vi "Remakejh.vi"   [LabVIEW 2015]
uses:
  <vilib>/NXT/Block Support/NXT_InputPort.ctl
  <vilib>/NXT/Block Support/NXT_OutputPort.ctl
  <vilib>/NXT/Dual Mode Library/Sensors/Light_On.vi
  <vilib>/NXT/Dual Mode Library/Sensors/Sonar_cm.vi
  <vilib>/NXT/NXTIO Xnodes/NXTIONodeSubVIs/NXTMoveMotors.vi
  <vilib>/NXT/Dual Mode Library/Waits/Wait_Num(msec).vi
  <vilib>/NXT/Subs/LVHSConnector.ctl
  <vilib>/NXT/NXTIO Xnodes/AddressXNode/NXTIOAddress.xnode
  <vilib>/NXT/NXTIO Xnodes/NXTIOXNode/NXTIO.xnode
  <vilib>/NXT/LegoClasses/BrickReference/BrickReference.lvclass
types:
  T1 = typedef "NXT_OutputPort.ctl" = u8
  T2 = typedef "NXT_InputPort.ctl" = u32
  T3 = typedef "LVHSConnector.ctl" = refnum<class "BrickReference.lvclass">
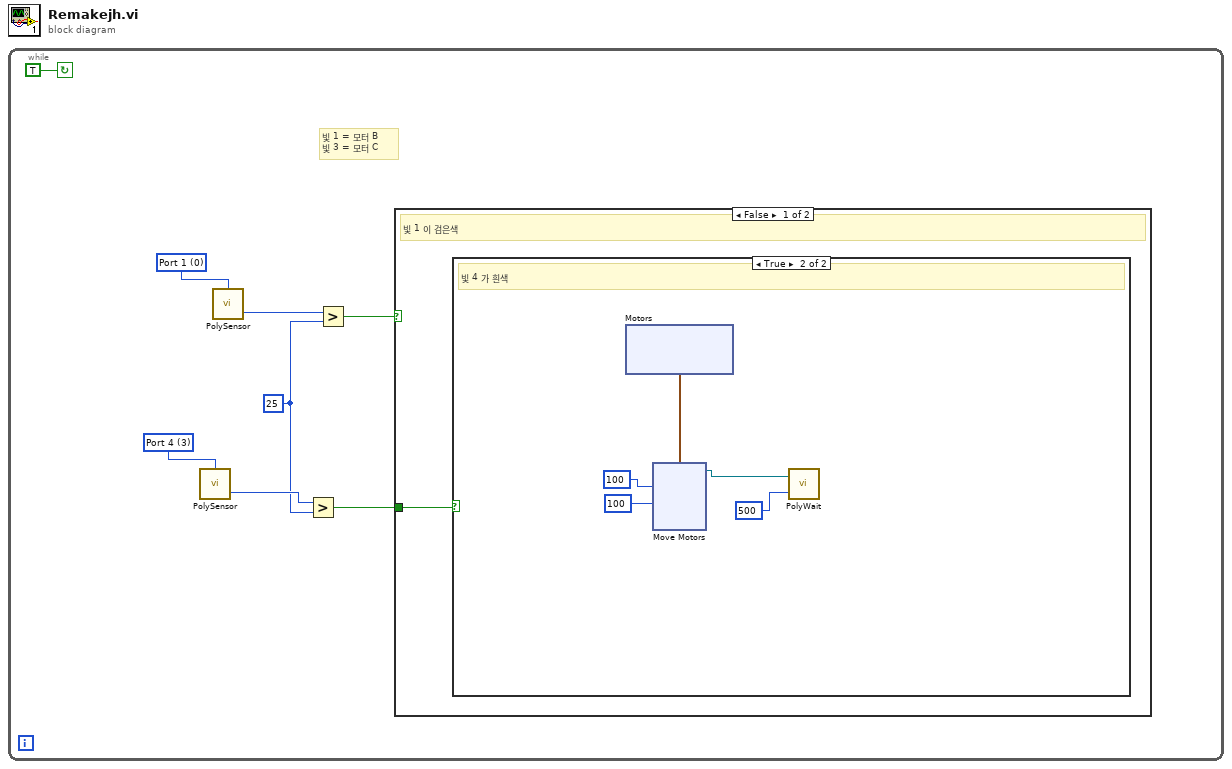
[diagram p0: block diagram]
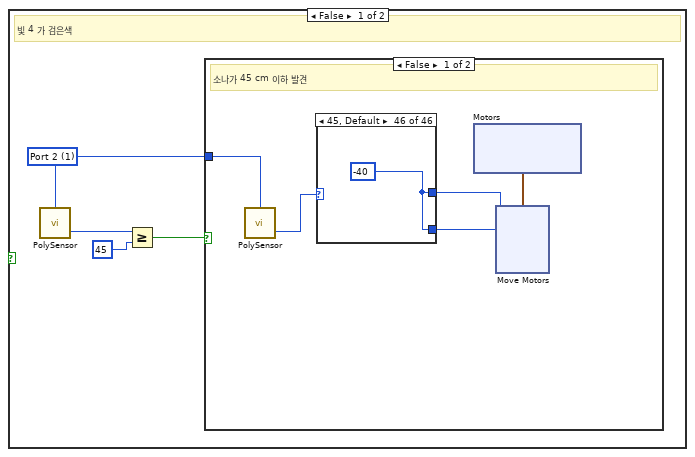
[diagram p2: hidden frame]
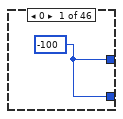
[diagram p3: hidden frame]
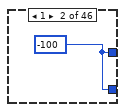
[diagram p4: hidden frame]
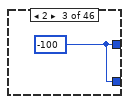
[diagram p5: hidden frame]
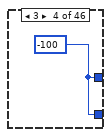
[diagram p6: hidden frame]
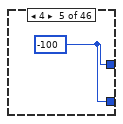
[diagram p7: hidden frame]
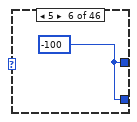
[diagram p8: hidden frame]
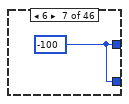
[diagram p9: hidden frame]
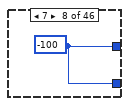
[diagram p10: hidden frame]
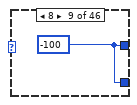
[diagram p11: hidden frame]
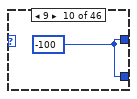
[diagram p12: hidden frame]
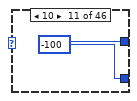
[diagram p13: hidden frame]
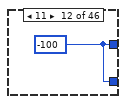
[diagram p14: hidden frame]
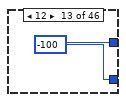
[diagram p15: hidden frame]
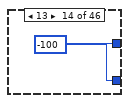
[diagram p16: hidden frame]
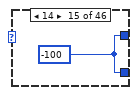
[diagram p17: hidden frame]
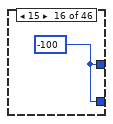
[diagram p18: hidden frame]
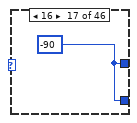
[diagram p19: hidden frame]
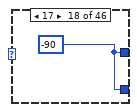
[diagram p20: hidden frame]
diagram:
  n1 = while {
    stop <- TRUE continue-if-true
    w1 = i16 25 ("y")
    w6 = T2 0 items=["Port 1", "Port 2", "Port 3", "Port 4"] ("Port (Port 3)")
    w5 = T2 3 items=["Port 1", "Port 2", "Port 3", "Port 4"] ("Port (Port 3)")
    # "빛 1 = 모터 B\n빛 3 = 모터 C"
    n2 = call-poly <vilib>:"PolySensor.vi"("Port (Port 3)"=w5) -> ("Scaled Value"=w7:i16)  [unwired: 2 in, 1 out]
    n3 = call-poly <vilib>:"PolySensor.vi"("Port (Port 3)"=w6) -> ("Scaled Value"=w8:i16)  [unwired: 2 in, 1 out]
    n4 = Greater?(x=w7, y=w1) -> (0:w3:bool)
    n5 = Greater?(x=w8, y=w1) -> (0:w4:bool)
    n6 = case shown="False" w4 {
      tunnel: w3 -> [w9 w122]
      frame False {
        # "빛 1 이 검은색"
        n7 = case shown="True" w9 {
          frame False {
            w10 = T2 1 items=["Port 1", "Port 2", "Port 3", "Port 4"] ("Port (Port 4)")
            # "빛 4 가 검은색"
            n8 = call-poly <vilib>:"PolySensor.vi"("Port (Port 4)"=w10) -> ("Distance (cm)"=w13:i16)  [unwired: 2 in, 1 out]
            n9 = Greater Or Equal?(x=w13, y=i16 45) -> (x >= y?=w11:bool)
            n10 = case shown="False" w11 {
              tunnel: w10 -> [w18 _]
              frame False {
                # "소나가 45 cm 이하 발견"
                n11 = call-poly <vilib>:"PolySensor.vi"("Port (Port 4)"=w18) -> ("Distance (cm)"=w17:i16)  [unwired: 2 in, 1 out]
                n12 = case shown="45, Default" w17 {
                  tunnel: [w28 w29 w30 w31 w32 w33 w34 w35 w36 w37 w38 w39 w40 w41 w42 w43 w44 w45 w46 w47 w48 w49 w50 w51 w52 w53 w54 w55 w56 w57 w58 w59 w60 w61 w62 w63 w64 w65 w66 w67 w68 w69 w70 w71 w72 w73] -> w15
                  tunnel: [w28 w29 w30 w31 w32 w33 w34 w35 w36 w37 w38 w39 w40 w41 w42 w43 w44 w45 w46 w47 w48 w49 w50 w51 w52 w53 w54 w55 w56 w57 w58 w59 w60 w61 w62 w63 w64 w65 w66 w67 w68 w69 w70 w71 w72 w73] -> w14
                  frame 0 {
                    w28 = i16 -100 ("y")
                  }
                  frame 1 {
                    w29 = i16 -100 ("y")
                  }
                  frame 2 {
                    w30 = i16 -100 ("y")
                  }
                  frame 3 {
                    w31 = i16 -100 ("y")
                  }
                  frame 4 {
                    w32 = i16 -100 ("y")
                  }
                  frame 5 {
                    w33 = i16 -100 ("y")
                  }
                  frame 6 {
                    w34 = i16 -100 ("y")
                  }
                  frame 7 {
                    w35 = i16 -100 ("y")
                  }
                  frame 8 {
                    w36 = i16 -100 ("y")
                  }
                  frame 9 {
                    w37 = i16 -100 ("y")
                  }
                  frame 10 {
                    w38 = i16 -100 ("y")
                  }
                  frame 11 {
                    w39 = i16 -100 ("y")
                  }
                  frame 12 {
                    w40 = i16 -100 ("y")
                  }
                  frame 13 {
                    w41 = i16 -100 ("y")
                  }
                  frame 14 {
                    w42 = i16 -100 ("y")
                  }
                  frame 15 {
                    w43 = i16 -100 ("y")
                  }
                  frame 16 {
                    w44 = i16 -90 ("y")
                  }
                  frame 17 {
                    w45 = i16 -90 ("y")
                  }
                  frame 18 {
                    w46 = i16 -90 ("y")
                  }
                  frame 19 {
                    w47 = i16 -90 ("y")
                  }
                  frame 20 {
                    w48 = i16 -90 ("y")
                  }
                  frame 21 {
                    w49 = i16 -80 ("y")
                  }
                  frame 22 {
                    w50 = i16 -80 ("y")
                  }
                  frame 23 {
                    w51 = i16 -80 ("y")
                  }
                  frame 24 {
                    w52 = i16 -80 ("y")
                  }
                  frame 25 {
                    w53 = i16 -80 ("y")
                  }
                  frame 26 {
                    w54 = i16 -70 ("y")
                  }
                  frame 27 {
                    w55 = i16 -70 ("y")
                  }
                  frame 28 {
                    w56 = i16 -70 ("y")
                  }
                  frame 29 {
                    w57 = i16 -70 ("y")
                  }
                  frame 30 {
                    w58 = i16 -70 ("y")
                  }
                  frame 31 {
                    w59 = i16 -60 ("y")
                  }
                  frame 32 {
                    w60 = i16 -60 ("y")
                  }
                  frame 33 {
                    w61 = i16 -60 ("y")
                  }
                  frame 34 {
                    w62 = i16 -60 ("y")
                  }
                  frame 35 {
                    w63 = i16 -60 ("y")
                  }
                  frame 36 {
                    w64 = i16 -50 ("y")
                  }
                  frame 37 {
                    w65 = i16 -50 ("y")
                  }
                  frame 38 {
                    w66 = i16 -50 ("y")
                  }
                  frame 39 {
                    w67 = i16 -50 ("y")
                  }
                  frame 40 {
                    w68 = i16 -50 ("y")
                  }
                  frame 41 {
                    w69 = i16 -40 ("y")
                  }
                  frame 42 {
                    w70 = i16 -40 ("y")
                  }
                  frame 43 {
                    w71 = i16 -40 ("y")
                  }
                  frame 44 {
                    w72 = i16 -40 ("y")
                  }
                  frame 45, Default {
                    w73 = i16 -40 ("y")
                  }
                }
                n13 = xnode "Motors"() -> ("Motor"=w16:cluster{"Port":T1, "Port":T1})
                n14 = xnode "Move Motors"("Power/Speed 2"=w14, "Power/Speed 1"=w15, "Motors"=w16) -> ()  [unwired: 1 in, 1 out]
              }
              frame True {
                w81 = i16 200 ("y")
                w80 = i16 50 ("y")
                w79 = i16 -50 ("y")
                # "소나가 45 cm 이상 발견"
                n15 = xnode "Motors"() -> ("Motor"=w82:cluster{"Port":T1, "Port":T1})
                n16 = xnode "Move Motors"("Power/Speed 2"=w79, "Power/Speed 1"=w79, "Motors"=w82) -> ("NXT/EV3"=w78:T3)  [unwired: 1 in]
                n17 = call-poly <vilib>:"PolyWait.vi"("Time (100 msec)"=w81, "NXT/EV3"=w78) -> ("NXT/EV3"=w77:T3)  [unwired: 2 in]
                n18 = xnode "Move Motors"("Power/Speed 2"=w79, "Power/Speed 1"=w80, "Motors"=w82, "NXT/EV3"=w77) -> ("NXT/EV3"=w76:T3)
                n19 = call-poly <vilib>:"PolyWait.vi"("Time (100 msec)"=w81, "NXT/EV3"=w76) -> ("NXT/EV3"=w75:T3)  [unwired: 2 in]
                n20 = xnode "Move Motors"("Power/Speed 2"=w80, "Power/Speed 1"=w79, "Motors"=w82, "NXT/EV3"=w75) -> ("NXT/EV3"=w74:T3)
                n21 = call-poly <vilib>:"PolyWait.vi"("Time (100 msec)"=w81, "NXT/EV3"=w74) -> ()  [unwired: 2 in, 1 out]
              }
            }
          }
          frame True {
            # "빛 4 가 흰색"
            n22 = xnode "Motors"() -> ("Motor"=w112:cluster{"Port":T1, "Port":T1})
            n23 = xnode "Move Motors"("Power/Speed 2"=i16 100 ("y"), "Power/Speed 1"=i16 100 ("y"), "Motors"=w112) -> ("NXT/EV3"=w108:T3)  [unwired: 1 in]
            n24 = call-poly <vilib>:"PolyWait.vi"("Time (100 msec)"=i16 500 ("y"), "NXT/EV3"=w108) -> ()  [unwired: 2 in, 1 out]
          }
        }
      }
      frame True {
        # "빛1이 흰색"
        n25 = case shown="False" w122 {
          frame False {
            # "빛 4가 검은색"
            n26 = xnode "Motors"() -> ("Motor"=w127:cluster{"Port":T1, "Port":T1})
            n27 = xnode "Move Motors"("Power/Speed 2"=i16 100 ("y"), "Power/Speed 1"=i16 100 ("y"), "Motors"=w127) -> ("NXT/EV3"=w123:T3)  [unwired: 1 in]
            n28 = call-poly <vilib>:"PolyWait.vi"("Time (100 msec)"=i16 500 ("y"), "NXT/EV3"=w123) -> ()  [unwired: 2 in, 1 out]
          }
          frame True {
            w137 = i16 100 ("y")
            # "빛4가 흰색"
            n29 = xnode "Motors"() -> ("Motor"=w144:cluster{"Port":T1, "Port":T1})
            n30 = xnode "Move Motors"("Power/Speed 2"=w137, "Power/Speed 1"=w137, "Motors"=w144) -> ("NXT/EV3"=w143:T3)  [unwired: 1 in]
            n31 = call-poly <vilib>:"PolyWait.vi"("Time (100 msec)"=i16 500 ("y"), "NXT/EV3"=w143) -> ("NXT/EV3"=w142:T3)  [unwired: 2 in]
            n32 = xnode "Move Motors"("Power/Speed 2"=w137, "Power/Speed 1"=i16 -100 ("y"), "Motors"=w144, "NXT/EV3"=w142) -> ("NXT/EV3"=w141:T3)
            n33 = call-poly <vilib>:"PolyWait.vi"("Time (100 msec)"=i16 700 ("y"), "NXT/EV3"=w141) -> ()  [unwired: 2 in, 1 out]
          }
        }
      }
    }
  }
